vi "Is Element Conversion Required.vi"(1 "element metadata":T1={"Field Name"="", "Embedded Message Name"="", "Protobuf Index"=1, "MessageElementType"=enum."StringValue", "Repeated"=FALSE, "Is in Oneof"=FALSE, "Oneof Container Name"=""}) -> (0 "conversion required":bool)   [LabVIEW 2019, in "gRPC Template Creation Utility.lvlib"]
uses:
  gRPC Template Creation Utility.lvlib
  TypeDefs/Message Element Metadata (Scripting).ctl
  TypeDefs/Message Element Type.ctl
  <vilib>/gRPC/LabVIEW gRPC Library/grpc-lvsupport-release.lvlib
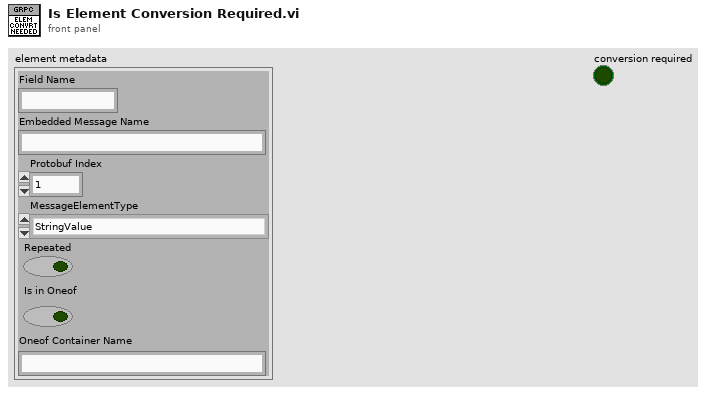
[diagram p1: front panel]
types:
  T1 = typedef "gRPC Template Creation Utility.lvlib/Message Element Metadata (Scripting).ctl" = cluster{"Field Name":string, "Embedded Message Name":string, "Protobuf Index":i32, "MessageElementType":T2, "Repeated":bool, "Is in Oneof":bool, "Oneof Container Name":string}
  T2 = typedef "gRPC Template Creation Utility.lvlib/Message Element Type.ctl" = enum32{"Int32Value", "FloatValue", "DoubleValue", "BoolValue", "StringValue", "MessageValue", "Int64Value", "UInt32Value", "UInt64Value", "EnumValue", "Bytes", "Fixed64", "Fixed32", "SFixed64", "SFixed32", "SInt64", "SInt32"}
  T3 = typedef "grpc-lvsupport-release.lvlib/Well Known Types.ctl" = enum32{"None", "Double2DArray", "String2DArray"}
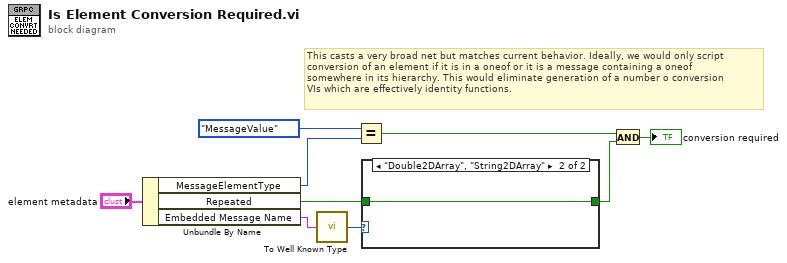
[diagram p0: block diagram]
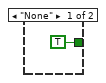
[diagram p2: hidden frame]
diagram:
  # "This casts a very broad net but matches current behavior. Ideally, we would only script\nconversion of an element if it is in a oneof or it is a message containing a oneof\nsomewhere in its hierarchy. This would eliminate generation of a number o conversion\nVIs which are effectively identity functions."
  n1 = Unbundle By Name("element metadata") -> ("MessageElementType"=w8:T2, "Repeated"=w3:bool, "Embedded Message Name"=w2:string)
  n2 = call <vilib>:"To Well Known Type.vi"("message name"=w2) -> ("well known type"=w1:T3)
  n3 = Equal?(x=Message_Element_Type."MessageValue", y=w8) -> (x = y?=w6:bool)
  n4 = case shown="\"Double2DArray\", \"String2DArray\"" w1 {
    tunnel: w3 -> [_ w11]
    tunnel: [TRUE w11] -> w5
    frame "None" {
    }
    frame "Double2DArray", "String2DArray" {
    }
  }
  n5 = And(x=w6, y=w5) -> (x .and. y?=→"conversion required":bool)
